vi "Harmonics MSMT Re-Configure SA Pin.vi"(8 "error in (no error)":errorcluster, 10 "Original SA Pin":string, 11 "Harmonics in":refnum<class "Harmonics.lvclass">) -> (0 "error out":errorcluster, 3 "Harmonics out":refnum<class "Harmonics.lvclass">)   [LabVIEW 2018, in "Harmonics.lvlib" / "Harmonics.lvclass"]
uses:
  Harmonics.lvclass
  C:/Sequence Automation/Plugins/Measurement Interface.lvlibp/Measurement Interface.lvclass
  Plugins/Measurement Interface.lvlibp/Private Methods/Measurement Parameters/Read Measurement Parameters.vi
  Plugins/Measurement Interface.lvlibp/Private Methods/Measurement Parameters/Write Measurement Parameters.vi
  Plugins/String Database.lvlibp/String Database.lvclass
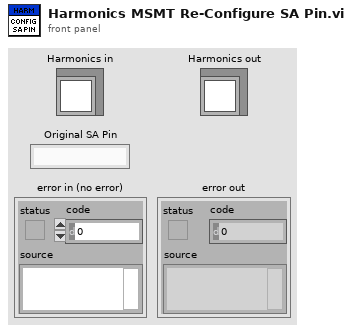
[diagram p1: front panel]
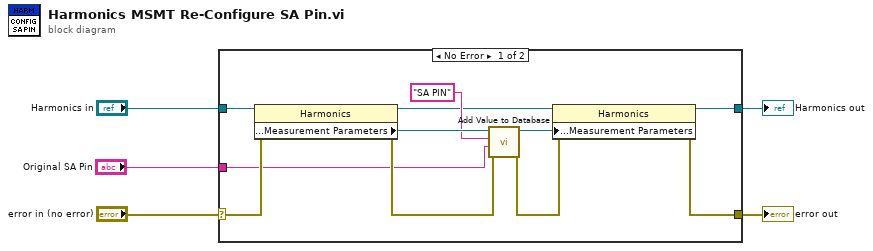
[diagram p0: block diagram]
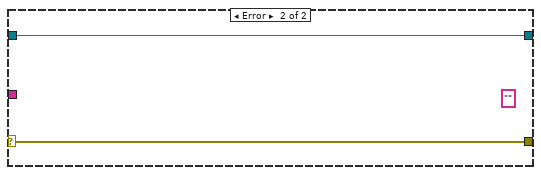
[diagram p2: hidden frame]
diagram:
  n1 = case shown="No Error" "error in (no error)" {
    selector: "error in (no error)" -> [w16 w18]
    tunnel: [w10 w18] -> w4
    tunnel: [w8 w17] -> w2
    tunnel: "Harmonics in" -> [w15 w17]
    tunnel: "Original SA Pin" -> [w6 _]
    frame No Error {
      n2 = property class="Harmonics"(reference=w15, error in=w16) -> (reference out=w9:refnum<class "Harmonics.lvclass">, error out=w13:errorcluster, "Protected Methods:Measurement Parameters"=w14:refnum<class "String Database.lvclass">)
      n3 = call "Add Value to Database.vi"("error in (no error)"=w13, "Entry Value"=w6, "Entry Name"="SA PIN", "Dictionary In"=w14) -> ("error out"=w11:errorcluster, "Dictionary Out"=w7:refnum<class "String Database.lvclass">)  [unwired: 5 in, 1 out]
      n4 = property class="Harmonics"(reference=w9, error in=w11, "Protected Methods:Measurement Parameters"=w7) -> (reference out=w8:refnum<class "Harmonics.lvclass">, error out=w10:errorcluster)
    }
    frame Error {
      (unwired) "" ("Entry Value")
    }
  }
  "error out" <- w4
  "Harmonics out" <- w2
